vi "Enqueue.vi"(0 "Queue Names In":string[](array[string]), 1 "Enqueue Type(Enqueue)":T2=enum."Enqueue", 5 "Message":string, 7 "Message Data":variant, 9 "Class":refnum<class "SensorBase.lvclass">, 11 "error in (no error)":errorcluster, 12 "EnqueueType (QMH)":T1, 13 "Create Queue? (F)":bool) -> (4 "MessageQueue":refnum<queue>, 6 "Queue Names Out":string[](array[string]), 15 "error out":errorcluster)   [LabVIEW 2018, in "SensorPlugins.lvlib"]
doc: "This VI places an element in the queue or deletes the existing element form the queue and places a new element in the queue."
uses:
  SensorPlugins.lvlib
  clMessage.ctl
  SensorBaseClass/SensorBase.lvclass
  EnqueueType.ctl
  QueueType.ctl
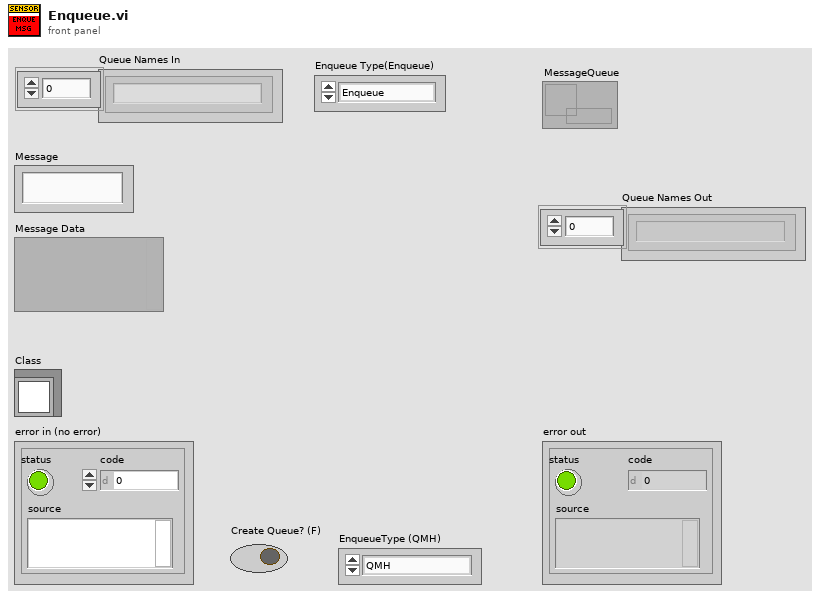
[diagram p1: front panel]
types:
  T1 = typedef "SensorPlugins.lvlib/QueueType.ctl" = enum16{"QMH", "Class ", "SP"}
  T2 = typedef "SensorPlugins.lvlib/EnqueueType.ctl" = enum16{"EnqueueAtFront", "Enqueue", "Lossy Enqueue"}
  T3 = typedef "SensorPlugins.lvlib/clMessage.ctl" = cluster{"Message":string, "Message Data":variant, "Class":refnum<class "SensorBase.lvclass">}
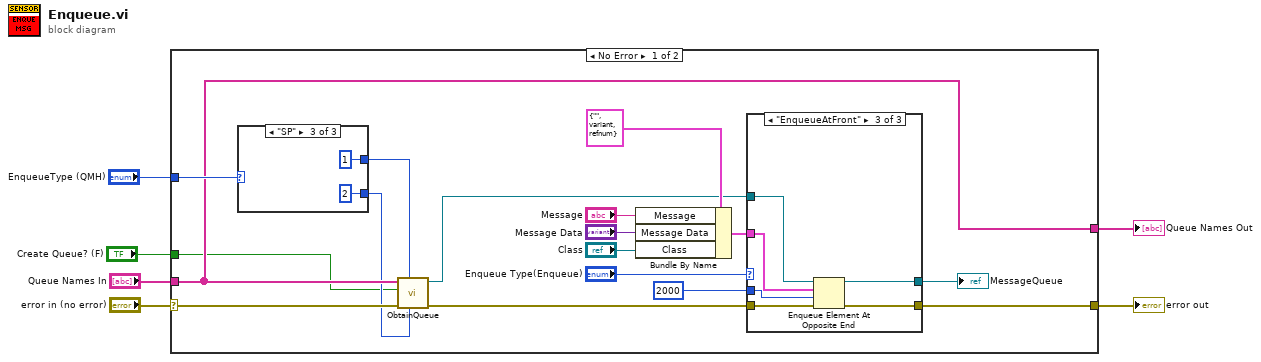
[diagram p0: block diagram]
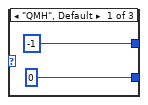
[diagram p2: hidden frame]
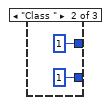
[diagram p3: hidden frame]
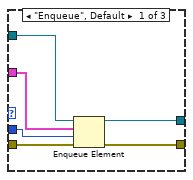
[diagram p4: hidden frame]
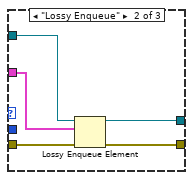
[diagram p5: hidden frame]
diagram:
  n1 = case shown="No Error" "error in (no error)" {
    selector: "error in (no error)" -> [w14 w48]
    tunnel: [w17 w48] -> w6
    tunnel: "Queue Names In" -> [w12 w47]
    tunnel: "EnqueueType (QMH)" -> [w15 _]
    tunnel: [w12 w47] -> w2
    tunnel: "Create Queue? (F)" -> [w7 _]
    frame No Error {
      n2 = case shown="\"SP\"" w15 {
        tunnel: [-1 ("max queue size (-1, unlimited)") 1 ("max queue size (-1, unlimited)") 1 ("max queue size (-1, unlimited)")] -> w13
        tunnel: [0 ("Queue Name Index (0) 2") 1 ("Queue Name Index (0) 2") 2 ("Queue Name Index (0) 2")] -> w11
        frame "QMH", Default {
        }
        frame "Class " {
        }
        frame "SP" {
        }
      }
      n3 = call "ObtainQueue.vi"("Queue Name Index"=w11, "max queue size (-1, unlimited)"=w13, "error in (no error)"=w14, "Create Queue? (F)"=w7, "Queue Names"=w12) -> ("error out"=w9:errorcluster, "MessageQueue"=w10:refnum<queue>)  [unwired: 5 in]
      n4 = Bundle By Name(cluster=T3 {"Message"="", "Message Data"=variant, "Class"=refnum} ("clMessage"), "Message"="Message", "Message Data"="Message Data", "Class"="Class") -> (w22:T3)
      n5 = case shown="\"EnqueueAtFront\"" "Enqueue Type(Enqueue)" {
        tunnel: w22 -> [w35 w37 w45]
        tunnel: w10 -> [w34 w40 w43]
        tunnel: [w33 w38 w42] -> w19
        tunnel: [w32 w39 w44] -> w17
        tunnel: w9 -> [w31 w36 w46]
        tunnel: 2000 ("timeout in ms (-1)") -> [w30 _ w41]
        frame "Enqueue", Default {
          n6 = Enqueue Element(queue=w34, element=w35, timeout in ms (-1)=w30, error in (no error)=w31) -> (queue out=w33:refnum<queue>, error out=w32:errorcluster)  [unwired: 1 out]
        }
        frame "Lossy Enqueue" {
          n7 = Lossy Enqueue Element(queue=w40, element=w37, error in (no error)=w36) -> (queue out=w38:refnum<queue>, error out=w39:errorcluster)  [unwired: 2 out]
        }
        frame "EnqueueAtFront" {
          n8 = Enqueue Element At Opposite End(queue=w43, element=w45, timeout in ms (-1)=w41, error in (no error)=w46) -> (queue out=w42:refnum<queue>, error out=w44:errorcluster)  [unwired: 1 out]
        }
      }
      "MessageQueue" <- w19
    }
    frame Error {
    }
  }
  "error out" <- w6
  "Queue Names Out" <- w2
